vi "Parse Response JSON.vi"(8 "error in (no error)":errorcluster, 10 "Response JSON":string, 11 "RToggleStream in":refnum<class "RToggleStream.lvclass">) -> (0 "error out":errorcluster, 3 "RToggleStream out":refnum<class "RToggleStream.lvclass">)   [LabVIEW 2020, in "obs-websocket.lvlib" / "RToggleStream.lvclass"]
uses:
  RToggleStream.lvclass
  RToggleStream.lvclass/RToggleStream.ctl
  <vilib>/IlluminatedG/lv-web-crypto/lv-json/JSON/JSON.lvlib
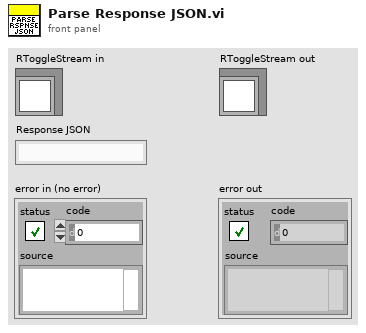
[diagram p1: front panel]
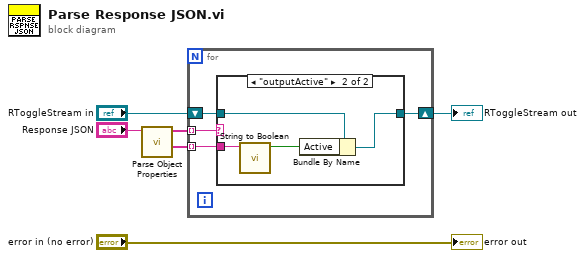
[diagram p0: block diagram]
diagram:
  n1 = call <vilib>:"Parse Object Properties.vi"("JSON String"="Response JSON") -> ("Values"=w3:string[], "Keys"=w4:string[])  [unwired: 7 in, 2 out]
  n2 = for {
    tunnel: w4 -> [w10] mode=indexing
    tunnel: w3 -> [w7] mode=indexing
    shift-right: [w8] -> w1
    shift-left: "RToggleStream in" -> [w9]
    n3 = case shown="\"outputActive\"" w10 {
      tunnel: w9 -> [w11 w15]
      tunnel: [w11 w14] -> w8
      tunnel: w7 -> [_ w13]
      frame Default {
      }
      frame "outputActive" {
        n4 = call <vilib>:"String to Boolean.vi"("Bool String"=w13) -> ("Boolean"=w12:bool)  [unwired: 10 in]
        n5 = Bundle By Name(cluster=w15, "Active"=w12) -> (w14:refnum<class "RToggleStream.lvclass">)
      }
    }
  }
  "RToggleStream out" <- w1
  "error out" <- "error in (no error)"
